vi "Start Timed Scan.vi"(0 "Notifier Name":string, 11 "Error In":errorcluster) -> (4 "Notifier Name Dup":string, 8 "Running":bool, 15 "Error Out":errorcluster)   [LabVIEW 2020]
uses:
  3 Mirror Scan Type Defs/3 Mirror Scan Note Type.ctl
  3 Mirror Scan Type Defs/3 Mirror Scan Actions.ctl
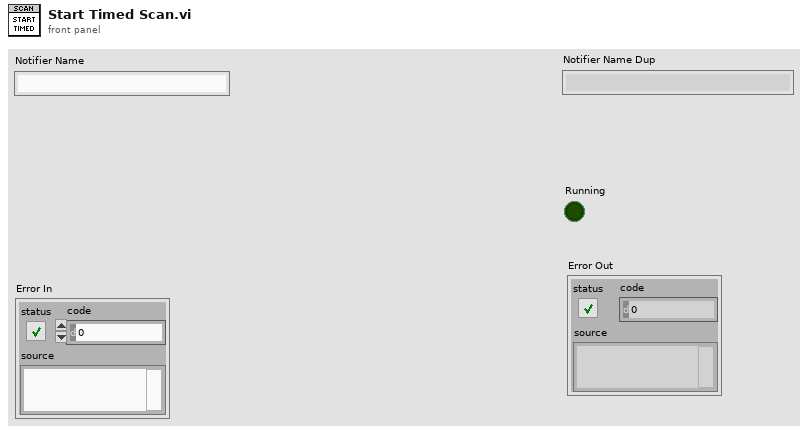
[diagram p1: front panel]
types:
  T1 = typedef "3 Mirror Scan Note Type.ctl" = cluster{"Actions":T2, "Global Rectangle":i32[], "Running":bool, "Scan Frequency (Hz)":dbl, "Scan Time (s)":dbl}
  T2 = typedef "3 Mirror Scan Actions.ctl" = enum16{"Idle", "Scan Timed", "Scan Live", "Convert ROI", "Run Scan", "Exit Loop", "Quit"}
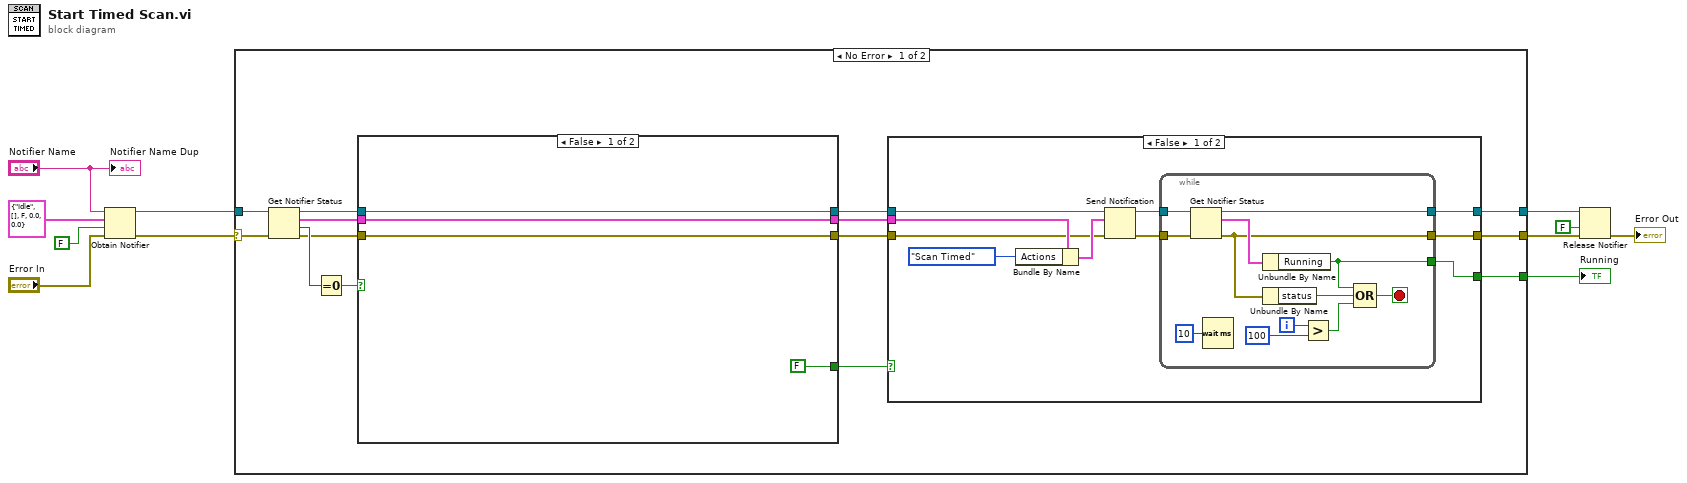
[diagram p0: block diagram]
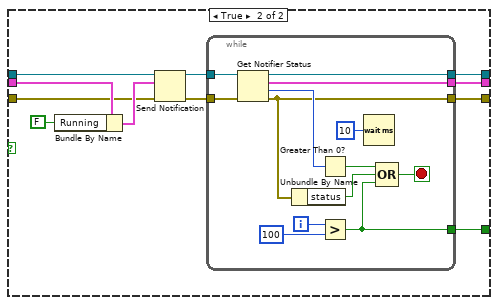
[diagram p2: hidden frame]
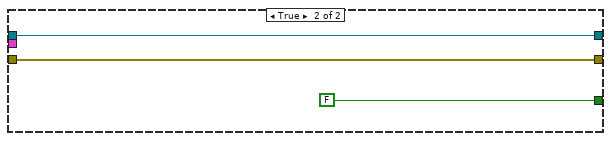
[diagram p3: hidden frame]
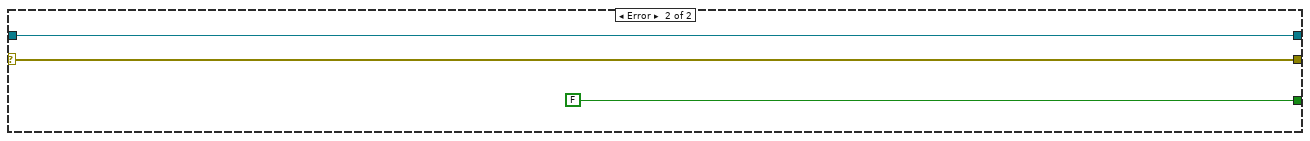
[diagram p4: hidden frame]
diagram:
  n1 = Obtain Notifier(name (unnamed)="Notifier Name", notification data type=T1 {"Actions"=enum."Idle", "Global Rectangle"=[], "Running"=FALSE, "Scan Frequency (Hz)"=0.0, "Scan Time (s)"=0.0} ("3 Mirror Notifier"), create if not found? (T)=FALSE, error in (no error)="Error In") -> (notifier out=w7:refnum<notifier>, error out=w8:errorcluster)  [unwired: 1 out]
  n2 = case shown="No Error" w8 {
    selector: w8 -> [w24 w80]
    tunnel: w7 -> [w25 w81]
    tunnel: [w23 w81] -> w5
    tunnel: [w22 w80] -> w3
    tunnel: [w21 FALSE] -> w1
    frame No Error {
      n3 = Get Notifier Status(notifier=w25, error in (no error)=w24) -> (notifier out=w19:refnum<notifier>, current notification=w20:T1, # waiting=w18:i32, error out=w17:errorcluster)  [unwired: 1 out]
      n4 = Equal To 0?(x=w18) -> (x = 0?=w16:bool)
      n5 = case shown="False" w16 {
        tunnel: w20 -> [w28 w40]
        tunnel: w19 -> [w29 w38]
        tunnel: w17 -> [w26 w36]
        tunnel: [FALSE w33] -> w15
        tunnel: [w29 w32] -> w14
        tunnel: [w28 w31] -> w13
        tunnel: [w26 w30] -> w12
        frame False {
        }
        frame True {
          n6 = Bundle By Name(cluster=w40, "Running"=FALSE) -> (w37:T1)
          n7 = Send Notification(notification=w37, notifier=w38, error in (no error)=w36) -> (notifier out=w35:refnum<notifier>, error out=w34:errorcluster)
          n8 = while {
            tunnel: w35 -> [w53]
            tunnel: w34 -> [w52]
            tunnel: [w45] -> w32
            tunnel: [w44] -> w33
            tunnel: [w43] -> w31
            tunnel: [w42] -> w30
            i -> [w50]
            stop <- w46 stop-if-true
            n9 = Get Notifier Status(notifier=w53, error in (no error)=w52) -> (notifier out=w45:refnum<notifier>, current notification=w43:T1, # waiting=w51:i32, error out=w42:errorcluster)  [unwired: 1 out]
            n10 = Unbundle By Name(w42) -> ("status"=w47:bool)
            n11 = Greater Than 0?(x=w51) -> (x > 0?=w48:bool)
            n12 = Greater?(x=w50, y=100) -> (0:w44:bool)
            n13 = Wait (ms)(milliseconds to wait=u32 10) -> ()  [unwired: 1 out]
            n14 = Compound Arithmetic op=OR(w48, w47, w44) -> (w46:bool)
          }
        }
      }
      n15 = case shown="False" w15 {
        tunnel: w12 -> [w59 w77]
        tunnel: w14 -> [w61 w78]
        tunnel: w13 -> [w63 _]
        tunnel: [w55 w78] -> w23
        tunnel: [w56 w77] -> w22
        tunnel: [w54 FALSE] -> w21
        frame False {
          n16 = Bundle By Name(cluster=w63, "Actions"=3_Mirror_Scan_Actions."Scan Timed") -> (w60:T1)
          n17 = Send Notification(notification=w60, notifier=w61, error in (no error)=w59) -> (notifier out=w58:refnum<notifier>, error out=w57:errorcluster)
          n18 = while {
            tunnel: w58 -> [w75]
            tunnel: w57 -> [w71]
            tunnel: [w66] -> w56
            tunnel: [w65] -> w55
            tunnel: [w64] -> w54
            i -> [w72]
            stop <- w67 stop-if-true
            n19 = Get Notifier Status(notifier=w75, error in (no error)=w71) -> (notifier out=w65:refnum<notifier>, current notification=w70:T1, error out=w66:errorcluster)  [unwired: 2 out]
            n20 = Wait (ms)(milliseconds to wait=u32 10) -> ()  [unwired: 1 out]
            n21 = Unbundle By Name(w70) -> ("Running"=w64:bool)
            n22 = Unbundle By Name(w66) -> ("status"=w69:bool)
            n23 = Greater?(x=w72, y=100) -> (0:w68:bool)
            n24 = Compound Arithmetic op=OR(w64, w69, w68) -> (w67:bool)
          }
        }
        frame True {
        }
      }
    }
    frame Error {
    }
  }
  "Running" <- w1
  n25 = Release Notifier(notifier=w5, force destroy? (F)=FALSE, error in (no error)=w3) -> (error out=→"Error Out":errorcluster)  [unwired: 2 out]
  "Notifier Name Dup" <- "Notifier Name"
